vi "GEA2 Script_Expected Response State.vi"(0 "Expected Response In":string, 11 "Error In":errorcluster) -> (2 "Response State":enum16{"None", "BIT"}(ring), 4 "Expected Response Out":string, 8 "Match Substring":string, 15 "Error Out":errorcluster)   [LabVIEW 2023]
uses:
  <vilib>/regexp/Match Regular Expression.xnode
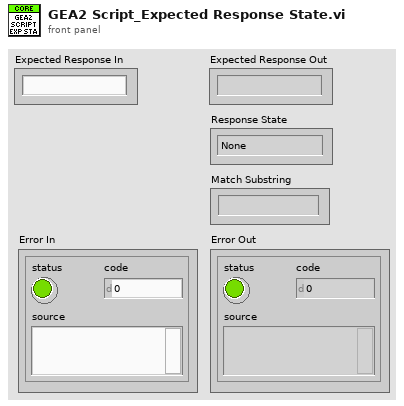
[diagram p1: front panel]
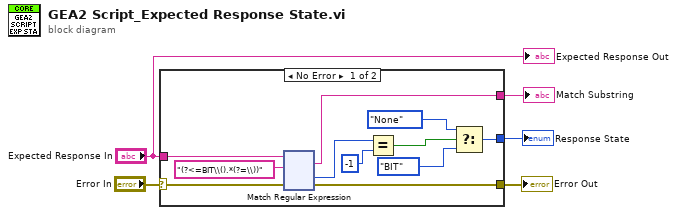
[diagram p0: block diagram]
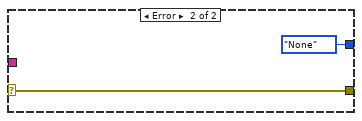
[diagram p2: hidden frame]
diagram:
  n1 = case shown="No Error" "Error In" {
    selector: "Error In" -> [w8 w135]
    tunnel: [w12 enum16{"None", "LED"}."None"] -> w5
    tunnel: "Expected Response In" -> [w10 _]
    tunnel: [w7 w135] -> w2
    tunnel: [w11 _] -> w1
    frame No Error {
      n2 = xnode "Match Regular Expression"("input string"=w10, "regular expression"="(?<=BIT\\().*(?=\\))", "error in"=w8) -> ("whole match"=w11:string, "offset past match"=w9:i32, "error out"=w7:errorcluster)  [unwired: 3 in, 2 out]
      n3 = Equal?(x=w9, y=-1) -> (x = y?=w14:bool)
      n4 = Select(t=enum16{"None", "BIT"}."None", s=w14, f=enum16{"None", "BIT"}."BIT") -> (s? t:f=w12:enum16{"None", "BIT"})
    }
    frame Error {
    }
  }
  "Response State" <- w5
  "Error Out" <- w2
  "Match Substring" <- w1
  "Expected Response Out" <- "Expected Response In"
